vi "List Tags By Type.vi"(8 "error in (no error)":errorcluster, 9 "NI Specific Type":T2, 10 "Broad Types":T1, 11 "Var Bus in":refnum<class "Multi_Bus.lvclass">) -> (0 "error out":errorcluster, 1 "Classes":refnum<class "Abs_Type.lvclass">[](array[class]), 2 "Tags":string[](array[string]), 3 "Var Bus out":refnum<class "Multi_Bus.lvclass">)   [LabVIEW 2021, in "Multi_Bus.lvclass"]
uses:
  Multi_Bus.lvclass
  <vilib>/Utility/Data Type/Type Definitions/Data Type.ctl
  Support/Broad Types.ctl
  Multi_Bus.lvclass/Multi_Bus.ctl
  <vilib>/TSA/Abstract Data Classes/Abs_Types/Numeric/Abs_Numeric.lvclass
  <vilib>/TSA/Abstract Data Classes/Abs_Types/Floating Point/Abs_Floating Point.lvclass
  <vilib>/TSA/Abstract Data Classes/Abs_Types/Boolean/Abs_Boolean.lvclass
  <vilib>/TSA/Abstract Data Classes/Abs_Types/String/Abs_String.lvclass
  <vilib>/TSA/Abstract Data Classes/Abs_Types/Integer/Abs_Integer.lvclass
  Properties/Read Var Map.vi
  <vilib>/TSA/Abstract Data Classes/Abs_Types/Type/Abs_Type.lvclass
  <vilib>/TSA/Abstract Data Classes/Abs_Types/Value/Abs_Value.lvclass
  C:/Program Files (x86)/National Instruments/LabVIEW 2021/vi.lib/TSA/Abstract Data Classes/Abs_Types/Type/Abs_Type.lvclass
  C:/Program Files (x86)/National Instruments/LabVIEW 2021/vi.lib/TSA/Abstract Data Classes/Abs_Types/Value/Abs_Value.lvclass
  <vilib>/Utility/Data Type/NI_Data Type.lvlib
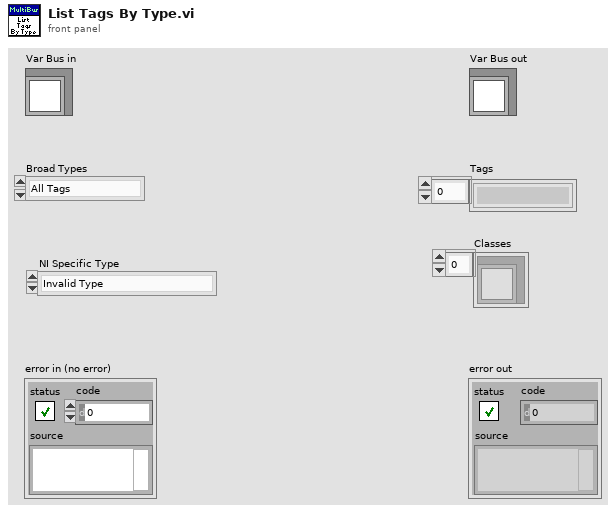
[diagram p1: front panel]
types:
  T1 = typedef "Multi_Bus.lvclass/Broad Types.ctl" = enum16{"All Tags", "NI Specific Type", "Boolean", "String", "Numeric", "Float", "Integer", "Collection", "All Value Types", "Non Value Types"}
  T2 = typedef "NI_Data Type.lvlib/Data Type.ctl" = enum8{"Invalid Type", "Void", "I8", "I16", "I32", "I64", "U8", "U16", "U32", "U64", "Single Float", "Double Float", "Extended Float", "Single Complex", "Double Complex", "Extended Complex", "Enum U8", "Enum U16", "Enum U32", "Enum U64", "Single Float With Unit", "Double Float With Unit", "Extended Float With Unit", "Single Complex with Unit", "Double Complex with Unit", "Extended Complex with Unit", "Boolean", "String", "Path", "Picture", "Tag", "Array", "Cluster", "Variant", "LV Variant", "Waveform", "Timestamp", "Digital Waveform", "Digital Data", "ExpressData", "Refnum", "External Data", "VI", "Poly VI", "LabVIEW Class Instance", "Fixed Point", "Set Collection", "Map Collection"}
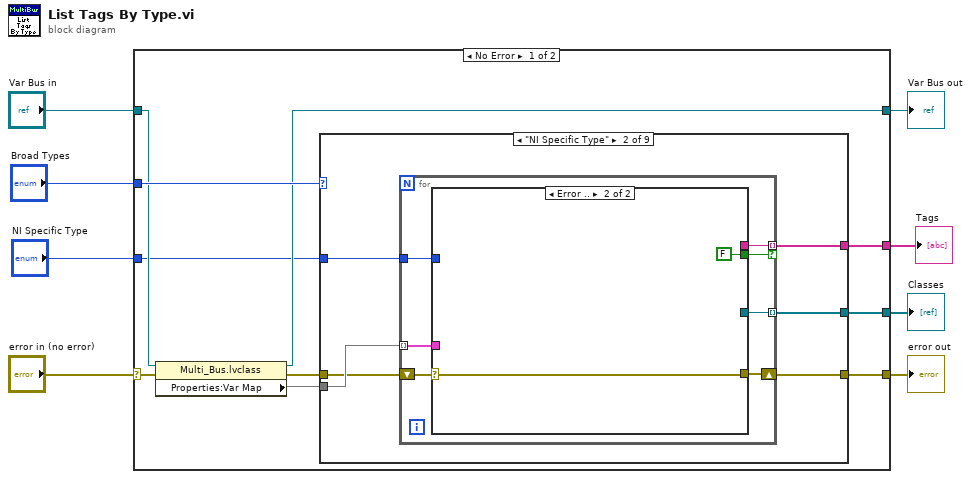
[diagram p0: block diagram]
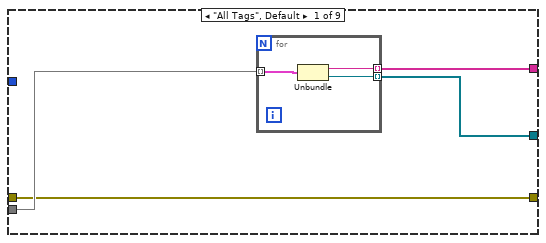
[diagram p2: hidden frame]
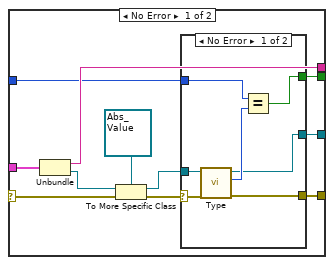
[diagram p3: hidden frame]
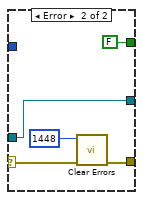
[diagram p4: hidden frame]
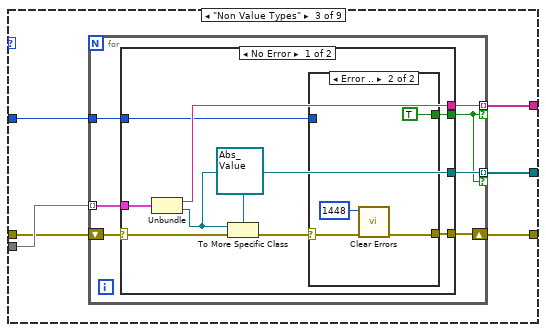
[diagram p5: hidden frame]
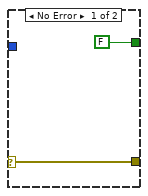
[diagram p6: hidden frame]
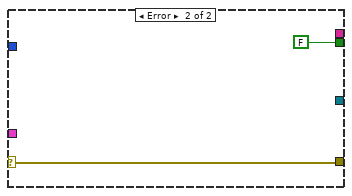
[diagram p7: hidden frame]
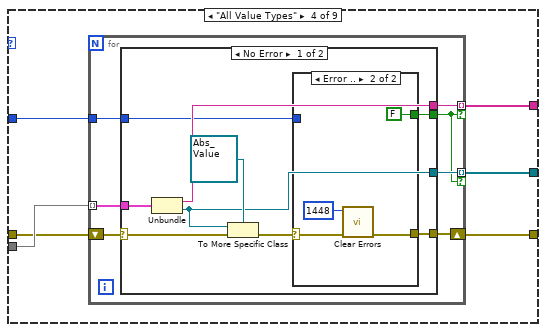
[diagram p8: hidden frame]
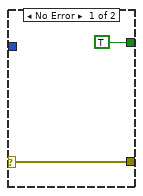
[diagram p9: hidden frame]
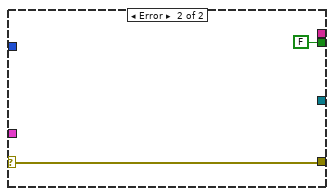
[diagram p10: hidden frame]
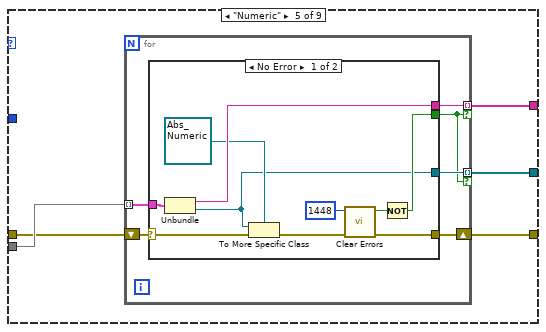
[diagram p11: hidden frame]
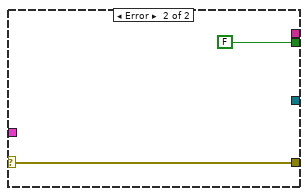
[diagram p12: hidden frame]
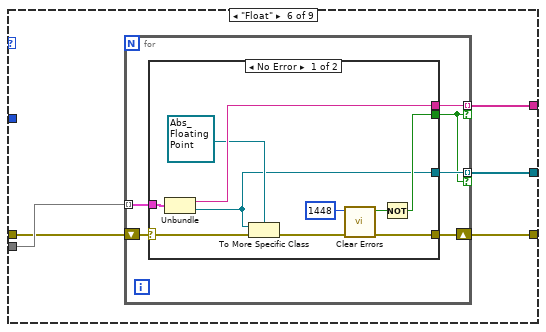
[diagram p13: hidden frame]
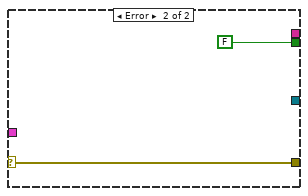
[diagram p14: hidden frame]
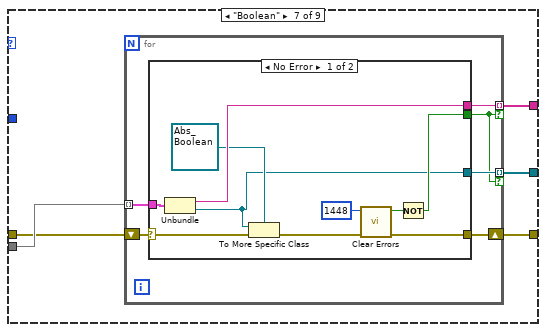
[diagram p15: hidden frame]
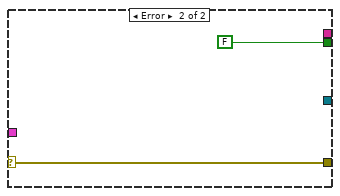
[diagram p16: hidden frame]
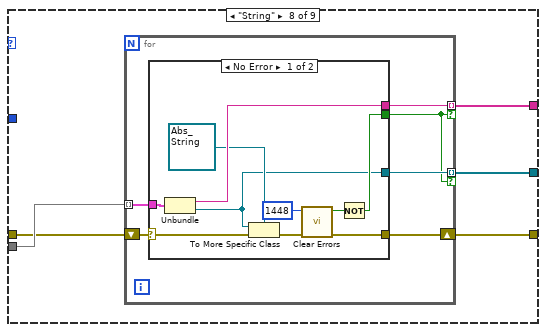
[diagram p17: hidden frame]
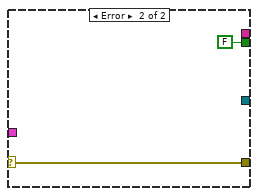
[diagram p18: hidden frame]
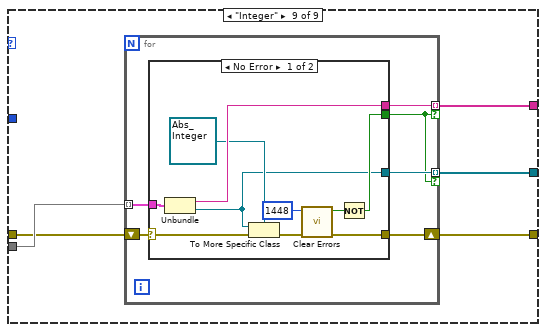
[diagram p19: hidden frame]
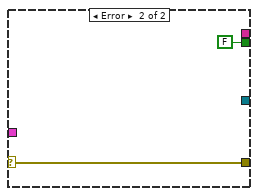
[diagram p20: hidden frame]
diagram:
  n1 = case shown="No Error" "error in (no error)" {
    selector: "error in (no error)" -> [w12 w240]
    tunnel: [w11 w240] -> w7
    tunnel: [w15 w239] -> w5
    tunnel: "Var Bus in" -> [w16 w239]
    tunnel: "Broad Types" -> [w18 _]
    tunnel: [w17 _] -> w3
    tunnel: "NI Specific Type" -> [w10 _]
    tunnel: [w9 _] -> w1
    frame No Error {
      n2 = property class="Multi_Bus.lvclass"(reference=w16, error in=w12) -> (reference out=w15:refnum<class "Multi_Bus.lvclass">, error out=w13:errorcluster, "Properties:Var Map"=w14:map{string, refnum<class "Abs_Type.lvclass">})
      n3 = case shown="\"NI Specific Type\"" w18 {
        tunnel: w13 -> [w20 w29 w67 w97 w126 w149 w172 w195 w218]
        tunnel: [w20 w27 w65 w95 w125 w148 w171 w194 w217] -> w11
        tunnel: [w22 w31 w69 w99 w128 w151 w174 w197 w220] -> w17
        tunnel: w14 -> [w21 w30 w68 w98 w127 w150 w173 w196 w219]
        tunnel: w10 -> [_ w28 w66 w96 _ _ _ _ _]
        tunnel: [w19 w26 w64 w94 w124 w147 w170 w193 w216] -> w9
        frame "All Tags", Default {
          n4 = for {
            tunnel: w21 -> [w25] mode=indexing
            tunnel: [w24] -> w22 mode=indexing
            tunnel: [w23] -> w19 mode=indexing
            n5 = Unbundle(w25) -> (w24:string, "Abs_Type.lvclass"=w23:refnum<class "Abs_Type.lvclass">)
          }
        }
        frame "NI Specific Type" {
          n6 = for {
            tunnel: w30 -> [w38] mode=indexing
            tunnel: [w37] -> w31 mode=indexing if=w34
            shift-right: [w36] -> w27
            shift-left: w29 -> [w33]
            tunnel: w28 -> [w35]
            tunnel: [w32] -> w26 mode=indexing
            n7 = case shown="Error .." w33 {
              selector: w33 -> [w44 w62]
              tunnel: w38 -> [w49 _]
              tunnel: [w48 _] -> w37
              tunnel: [w47 w62] -> w36
              tunnel: w35 -> [w46 _]
              tunnel: [w45 FALSE] -> w34
              tunnel: [w39 _] -> w32
              frame No Error {
                n8 = Unbundle(w49) -> (w48:string, "Abs_Type.lvclass"=w42:refnum<class "Abs_Type.lvclass">)
                n9 = To More Specific Class(target class=refnum<class "Abs_Value.lvclass"> refnum ("Abs_Value.lvclass"), reference=w42, error in=w44) -> (specific class reference=w40:refnum<class "Abs_Value.lvclass">, error out=w43:errorcluster)
                n10 = case shown="No Error" w43 {
                  selector: w43 -> [w52 w61]
                  tunnel: [w56 w60] -> w47
                  tunnel: w46 -> [w54 _]
                  tunnel: [w53 FALSE] -> w45
                  tunnel: w40 -> [w51 w57]
                  tunnel: [w50 w57] -> w39
                  frame No Error {
                    n11 = call-dynamic "Type.vi"("error in (no error)"=w52, "Element in"=w51) -> ("error out"=w56:errorcluster, "Type"=w55:T2, "Element out"=w50:refnum<class "Abs_Value.lvclass">)  [unwired: 7 in]
                    n12 = Equal?(x=w54, y=w55) -> (x = y?=w53:bool)
                  }
                  frame Error {
                    n13 = call <vilib>:"Clear Errors.vi"("error in (no error)"=w61, "specific error code to clear (0: all)"=1448) -> ("error out"=w60:errorcluster)  [unwired: 4 in, 1 out]
                  }
                }
              }
              frame Error {
              }
            }
          }
        }
        frame "Non Value Types" {
          n14 = for {
            tunnel: w68 -> [w76] mode=indexing
            tunnel: [w75] -> w69 mode=indexing if=w70
            shift-right: [w74] -> w65
            shift-left: w67 -> [w72]
            tunnel: w66 -> [w73]
            tunnel: [w71] -> w64 mode=indexing if=w70
            n15 = case shown="No Error" w72 {
              selector: w72 -> [w80 w92]
              tunnel: w76 -> [w85 _]
              tunnel: [w84 _] -> w75
              tunnel: [w83 w92] -> w74
              tunnel: w73 -> [w82 _]
              tunnel: [w81 FALSE] -> w70
              tunnel: [w77 _] -> w71
              frame No Error {
                n16 = Unbundle(w85) -> (w84:string, "Abs_Type.lvclass"=w77:refnum<class "Abs_Type.lvclass">)
                n17 = To More Specific Class(target class=refnum<class "Abs_Value.lvclass"> refnum ("Abs_Value.lvclass"), reference=w77, error in=w80) -> (error out=w79:errorcluster)  [unwired: 1 out]
                n18 = case shown="Error .." w79 {
                  selector: w79 -> [w87 w91]
                  tunnel: [w87 w90] -> w83
                  tunnel: w82 -> [_ _]
                  tunnel: [FALSE TRUE] -> w81
                  frame No Error {
                  }
                  frame Error {
                    n19 = call <vilib>:"Clear Errors.vi"("error in (no error)"=w91, "specific error code to clear (0: all)"=1448) -> ("error out"=w90:errorcluster)  [unwired: 4 in, 1 out]
                  }
                }
              }
              frame Error {
              }
            }
          }
        }
        frame "All Value Types" {
          n20 = for {
            tunnel: w98 -> [w106] mode=indexing
            tunnel: [w105] -> w99 mode=indexing if=w100
            shift-right: [w104] -> w95
            shift-left: w97 -> [w102]
            tunnel: w96 -> [w103]
            tunnel: [w101] -> w94 mode=indexing if=w100
            n21 = case shown="No Error" w102 {
              selector: w102 -> [w110 w122]
              tunnel: w106 -> [w115 _]
              tunnel: [w114 _] -> w105
              tunnel: [w113 w122] -> w104
              tunnel: w103 -> [w112 _]
              tunnel: [w111 FALSE] -> w100
              tunnel: [w107 _] -> w101
              frame No Error {
                n22 = Unbundle(w115) -> (w114:string, "Abs_Type.lvclass"=w107:refnum<class "Abs_Type.lvclass">)
                n23 = To More Specific Class(target class=refnum<class "Abs_Value.lvclass"> refnum ("Abs_Value.lvclass"), reference=w107, error in=w110) -> (error out=w109:errorcluster)  [unwired: 1 out]
                n24 = case shown="Error .." w109 {
                  selector: w109 -> [w117 w121]
                  tunnel: [w117 w120] -> w113
                  tunnel: w112 -> [_ _]
                  tunnel: [TRUE FALSE] -> w111
                  frame No Error {
                  }
                  frame Error {
                    n25 = call <vilib>:"Clear Errors.vi"("error in (no error)"=w121, "specific error code to clear (0: all)"=1448) -> ("error out"=w120:errorcluster)  [unwired: 4 in, 1 out]
                  }
                }
              }
              frame Error {
              }
            }
          }
        }
        frame "Numeric" {
          n26 = for {
            tunnel: w127 -> [w134] mode=indexing
            tunnel: [w133] -> w128 mode=indexing if=w129
            shift-right: [w131] -> w125
            shift-left: w126 -> [w132]
            tunnel: [w130] -> w124 mode=indexing if=w129
            n27 = case shown="No Error" w132 {
              selector: w132 -> [w142 w146]
              tunnel: w134 -> [w144 _]
              tunnel: [w143 _] -> w133
              tunnel: [w139 w146] -> w131
              tunnel: [w137 FALSE] -> w129
              tunnel: [w135 _] -> w130
              frame No Error {
                n28 = Unbundle(w144) -> (w143:string, "Abs_Type.lvclass"=w135:refnum<class "Abs_Type.lvclass">)
                n29 = To More Specific Class(target class=refnum<class "Abs_Numeric.lvclass"> refnum ("Abs_Numeric.lvclass"), reference=w135, error in=w142) -> (error out=w140:errorcluster)  [unwired: 1 out]
                n30 = call <vilib>:"Clear Errors.vi"("error in (no error)"=w140, "specific error code to clear (0: all)"=1448) -> ("error out"=w139:errorcluster, "specific error cleared?"=w138:bool)  [unwired: 4 in]
                n31 = Not(x=w138) -> (.not. x?=w137:bool)
              }
              frame Error {
              }
            }
          }
        }
        frame "Float" {
          n32 = for {
            tunnel: w150 -> [w157] mode=indexing
            tunnel: [w156] -> w151 mode=indexing if=w152
            shift-right: [w154] -> w148
            shift-left: w149 -> [w155]
            tunnel: [w153] -> w147 mode=indexing if=w152
            n33 = case shown="No Error" w155 {
              selector: w155 -> [w165 w169]
              tunnel: w157 -> [w167 _]
              tunnel: [w166 _] -> w156
              tunnel: [w163 w169] -> w154
              tunnel: [w161 FALSE] -> w152
              tunnel: [w158 _] -> w153
              frame No Error {
                n34 = Unbundle(w167) -> (w166:string, "Abs_Type.lvclass"=w158:refnum<class "Abs_Type.lvclass">)
                n35 = To More Specific Class(target class=refnum<class "Abs_Floating Point.lvclass"> refnum ("Abs_Floating Point.lvclass"), reference=w158, error in=w165) -> (error out=w164:errorcluster)  [unwired: 1 out]
                n36 = call <vilib>:"Clear Errors.vi"("error in (no error)"=w164, "specific error code to clear (0: all)"=1448) -> ("error out"=w163:errorcluster, "specific error cleared?"=w162:bool)  [unwired: 4 in]
                n37 = Not(x=w162) -> (.not. x?=w161:bool)
              }
              frame Error {
              }
            }
          }
        }
        frame "Boolean" {
          n38 = for {
            tunnel: w173 -> [w180] mode=indexing
            tunnel: [w179] -> w174 mode=indexing if=w175
            shift-right: [w177] -> w171
            shift-left: w172 -> [w178]
            tunnel: [w176] -> w170 mode=indexing if=w175
            n39 = case shown="No Error" w178 {
              selector: w178 -> [w188 w192]
              tunnel: w180 -> [w190 _]
              tunnel: [w189 _] -> w179
              tunnel: [w186 w192] -> w177
              tunnel: [w184 FALSE] -> w175
              tunnel: [w181 _] -> w176
              frame No Error {
                n40 = Unbundle(w190) -> (w189:string, "Abs_Type.lvclass"=w181:refnum<class "Abs_Type.lvclass">)
                n41 = To More Specific Class(target class=refnum<class "Abs_Boolean.lvclass"> refnum ("Abs_Boolean.lvclass"), reference=w181, error in=w188) -> (error out=w187:errorcluster)  [unwired: 1 out]
                n42 = call <vilib>:"Clear Errors.vi"("error in (no error)"=w187, "specific error code to clear (0: all)"=1448) -> ("error out"=w186:errorcluster, "specific error cleared?"=w185:bool)  [unwired: 4 in]
                n43 = Not(x=w185) -> (.not. x?=w184:bool)
              }
              frame Error {
              }
            }
          }
        }
        frame "String" {
          n44 = for {
            tunnel: w196 -> [w203] mode=indexing
            tunnel: [w202] -> w197 mode=indexing if=w198
            shift-right: [w200] -> w194
            shift-left: w195 -> [w201]
            tunnel: [w199] -> w193 mode=indexing if=w198
            n45 = case shown="No Error" w201 {
              selector: w201 -> [w211 w215]
              tunnel: w203 -> [w213 _]
              tunnel: [w212 _] -> w202
              tunnel: [w209 w215] -> w200
              tunnel: [w207 FALSE] -> w198
              tunnel: [w204 _] -> w199
              frame No Error {
                n46 = Unbundle(w213) -> (w212:string, "Abs_Type.lvclass"=w204:refnum<class "Abs_Type.lvclass">)
                n47 = To More Specific Class(target class=refnum<class "Abs_String.lvclass"> refnum ("Abs_String.lvclass"), reference=w204, error in=w211) -> (error out=w210:errorcluster)  [unwired: 1 out]
                n48 = call <vilib>:"Clear Errors.vi"("error in (no error)"=w210, "specific error code to clear (0: all)"=1448) -> ("error out"=w209:errorcluster, "specific error cleared?"=w208:bool)  [unwired: 4 in]
                n49 = Not(x=w208) -> (.not. x?=w207:bool)
              }
              frame Error {
              }
            }
          }
        }
        frame "Integer" {
          n50 = for {
            tunnel: w219 -> [w226] mode=indexing
            tunnel: [w225] -> w220 mode=indexing if=w221
            shift-right: [w223] -> w217
            shift-left: w218 -> [w224]
            tunnel: [w222] -> w216 mode=indexing if=w221
            n51 = case shown="No Error" w224 {
              selector: w224 -> [w234 w238]
              tunnel: w226 -> [w236 _]
              tunnel: [w235 _] -> w225
              tunnel: [w232 w238] -> w223
              tunnel: [w230 FALSE] -> w221
              tunnel: [w227 _] -> w222
              frame No Error {
                n52 = Unbundle(w236) -> (w235:string, "Abs_Type.lvclass"=w227:refnum<class "Abs_Type.lvclass">)
                n53 = To More Specific Class(target class=refnum<class "Abs_Integer.lvclass"> refnum ("Abs_Integer.lvclass"), reference=w227, error in=w234) -> (error out=w233:errorcluster)  [unwired: 1 out]
                n54 = call <vilib>:"Clear Errors.vi"("error in (no error)"=w233, "specific error code to clear (0: all)"=1448) -> ("error out"=w232:errorcluster, "specific error cleared?"=w231:bool)  [unwired: 4 in]
                n55 = Not(x=w231) -> (.not. x?=w230:bool)
              }
              frame Error {
              }
            }
          }
        }
      }
    }
    frame Error {
    }
  }
  "error out" <- w7
  "Var Bus out" <- w5
  "Tags" <- w3
  "Classes" <- w1
